vi "Get Settings.vi"(8 "error in (no error)":errorcluster, 11 "Configuration in":refnum<class "Configuration.lvclass">) -> (0 "error out":errorcluster, 2 "settings":T1, 3 "Configuration out":refnum<class "Configuration.lvclass">)   [LabVIEW 2017, in "DSF Core.lvlib" / "Configuration.lvclass"]
uses:
  Configuration.lvclass
  DSF Configuration API/Public/Controls/DSF Settings Info.ctl
  Configuration.lvclass/Configuration.ctl
  DSF Core.lvlib
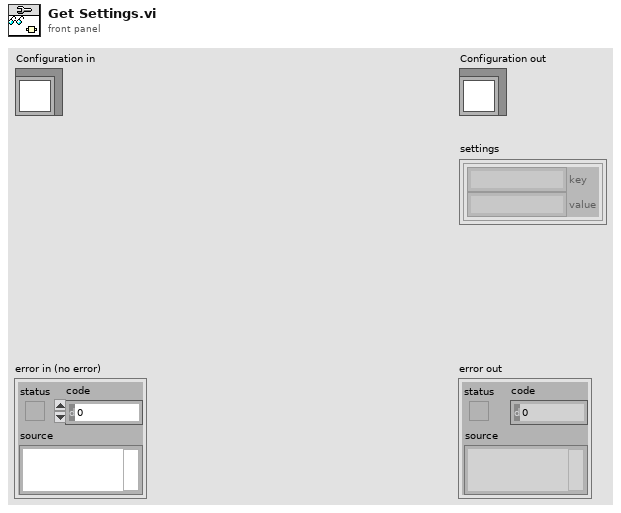
[diagram p1: front panel]
types:
  T1 = typedef "DSF Core.lvlib/DSF Settings Info.ctl" = cluster{"key":string, "value":string}[]
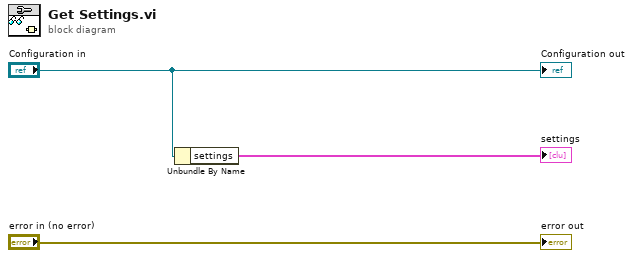
[diagram p0: block diagram]
diagram:
  n1 = Unbundle By Name("Configuration in") -> ("settings"=→"settings":T1)
  "error out" <- "error in (no error)"
  "Configuration out" <- "Configuration in"
